vi "ROI_IN_Check.vi"(8 "도형Y좌표":i32[](array[numeric]), 9 "도형X좌표":i32[](array[numeric]), 10 "LiDAR_Y":i32[](array[numeric]), 11 "LiDAR_X":i32[](array[numeric])) -> (0 "ROI_IN_Y":i32[](array[numeric]), 3 "ROI_IN_X":i32[](array[numeric]))   [LabVIEW 2019]
uses:
  <vilib>/Analysis/geometry.llb/Point in Polygon (Scalar).vi
  <vilib>/Analysis/NI_AAL_Geometry.lvlib
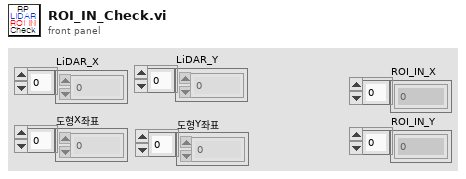
[diagram p1: front panel]
types:
  T1 = typedef "NI_AAL_Geometry.lvlib/Point in Polygon Position.ctl" = u16
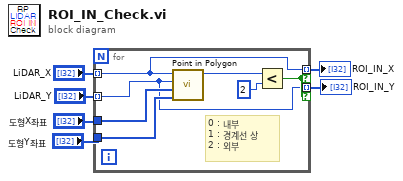
[diagram p0: block diagram]
diagram:
  n1 = for {
    tunnel: "LiDAR_Y" -> [w7] mode=indexing
    tunnel: "LiDAR_X" -> [w8] mode=indexing
    tunnel: "도형X좌표" -> [w13]
    tunnel: "도형Y좌표" -> [w12]
    tunnel: [w8] -> w2 mode=indexing if=w9
    tunnel: [w7] -> w1 mode=indexing if=w9
    # "0 : 내부\n1 : 경계선 상\n2 : 외부"
    n2 = call-poly <vilib>:"Point in Polygon.vi"("Polygon Y"=w12, "Polygon X"=w13, "y"=w7, "x"=w8) -> ("position"=w11:T1)  [unwired: 6 in, 1 out]
    n3 = Less?(x=w11, y=u16 2) -> (x < y?=w9:bool)
  }
  "ROI_IN_X" <- w2
  "ROI_IN_Y" <- w1
